vi "Calculate Intersection.vi"(0 "Coordinate Array":cluster{"X":dbl, "Y":dbl}[](array[cluster])=[{"X"=17.695146305622988, "Y"=13.693373640688556}, {"X"=17.43433821214924, "Y"=13.745589252995408}, {"X"=17.162615396419707, "Y"=13.800431502574536}, {"X"=16.880666961571364, "Y"=13.857854049761876}, {"X"=16.589182010741155, "Y"=13.917810554893407}, {"X"=16.288849647066037, "Y"=13.980254678305073}, {"X"=15.98035897368297, "Y"=14.045140080332846}, {"X"=15.664399093728898, "Y"=14.112420421312695}, {"X"=15.341659110340789, "Y"=14.182049361580557}, {"X"=15.012828126655597, "Y"=14.253980561472414}, {"X"=14.678595245810266, "Y"=14.328167681324217}, {"X"=14.339649570941765, "Y"=14.404564381471928}, {"X"=13.996680205187042, "Y"=14.483124322251506}, {"X"=13.650376251683053, "Y"=14.563801163998928}, {"X"=13.301426813566753, "Y"=14.646548567050132}, {"X"=12.950520993975104, "Y"=14.73132019174109}, {"X"=12.598347896045052, "Y"=14.818069698407761}, {"X"=12.245596622913556, "Y"=14.906750747386106}, {"X"=11.892956277717579, "Y"=14.997316999012082}, {"X"=11.541115963594061, "Y"=15.089722113621658}, {"X"=11.190764783679967, "Y"=15.183919751550793}, {"X"=10.842591841112258, "Y"=15.279863573135437}, {"X"=10.497286239027877, "Y"=15.377507238711566}, {"X"=10.155537080563787, "Y"=15.47680440861513}, {"X"=9.81803346885694, "Y"=15.577708743182097}, {"X"=9.485464507044295, "Y"=15.680173902748418}, {"X"=9.158519298262807, "Y"=15.78415354765006}, {"X"=8.837886945649426, "Y"=15.889601338222992}, {"X"=8.524256552341113, "Y"=15.99647093480316}, {"X"=8.21831722147482, "Y"=16.104715997726533}, {"X"=7.920758056187506, "Y"=16.21429018732907}, {"X"=7.6322681596161255, "Y"=16.325147163946735}, {"X"=7.3535366348976305, "Y"=16.437240587915483}, {"X"=7.0852525851689805, "Y"=16.55052411957128}, {"X"=6.82810511356713, "Y"=16.66495141925008}, {"X"=6.58278332322903, "Y"=16.78047614728785}, {"X"=6.3499763172916435, "Y"=16.89705196402055}, {"X"=6.13037319889192, "Y"=17.014632529784137}, {"X"=5.924663071166817, "Y"=17.13317150491458}, {"X"=5.733535037253291, "Y"=17.252622549747834}, {"X"=5.557678200288295, "Y"=17.372939324619853}, {"X"=5.397781663408787, "Y"=17.494075489866614}, {"X"=5.25453452975172, "Y"=17.61598470582406}, {"X"=5.128625902454051, "Y"=17.738620632828166}, {"X"=5.020744884652735, "Y"=17.861936931214885}], 1 "Enum":enum16{"Horizontal", "Vertical"}(ring), 3 "Vertical X":dbl=9.0, 4 "Horizontal Y":dbl=15.0) -> (5 "Intersection":bool=TRUE, 6 "Horizontal X":dbl=11.88266096329118, 7 "Vertical Y":dbl=15.83628649564717, 8 "XY Graph":cluster{dbl[], dbl[]}[](graph)=[{[5.020744884652735, 5.128625902454051, 5.25453452975172, 5.397781663408787, 5.557678200288295, 5.733535037253291, 5.924663071166817, 6.13037319889192, 6.3499763172916435, 6.58278332322903, 6.82810511356713, 7.0852525851689805, 7.3535366348976305, 7.6322681596161255, 7.920758056187506, 8.21831722147482, 8.524256552341113, 8.837886945649426, 9.158519298262807, 9.485464507044295, 9.81803346885694, 10.155537080563787, 10.497286239027877, 10.842591841112258, 11.190764783679967, 11.541115963594061, 11.892956277717579, 12.245596622913556, 12.598347896045052, 12.950520993975104, 13.301426813566753, 13.650376251683053, 13.996680205187042, 14.339649570941765, 14.678595245810266, 15.012828126655597, 15.341659110340789, 15.664399093728898, 15.98035897368297, 16.288849647066037, 16.589182010741155, 16.880666961571364, 17.162615396419707, 17.43433821214924, 17.695146305622988], [17.861936931214885, 17.738620632828166, 17.61598470582406, 17.494075489866614, 17.372939324619853, 17.252622549747834, 17.13317150491458, 17.014632529784137, 16.89705196402055, 16.78047614728785, 16.66495141925008, 16.55052411957128, 16.437240587915483, 16.325147163946735, 16.21429018732907, 16.104715997726533, 15.99647093480316, 15.889601338222992, 15.78415354765006, 15.680173902748418, 15.577708743182097, 15.47680440861513, 15.377507238711566, 15.279863573135437, 15.183919751550793, 15.089722113621658, 14.997316999012082, 14.906750747386106, 14.818069698407761, 14.73132019174109, 14.646548567050132, 14.563801163998928, 14.483124322251506, 14.404564381471928, 14.328167681324217, 14.253980561472414, 14.182049361580557, 14.112420421312695, 14.045140080332846, 13.980254678305073, 13.917810554893407, 13.857854049761876, 13.800431502574536, 13.745589252995408, 13.693373640688556]}, {[9.0, 9.0, 9.0, 9.0, 9.0, 9.0, 9.0, 9.0, 9.0, 9.0, 9.0, 9.0, 9.0, 9.0, 9.0, 9.0, 9.0, 9.0, 9.0, 9.0, 9.0, 9.0, 9.0, 9.0, 9.0, 9.0, 9.0, 9.0, 9.0, 9.0, 9.0, 9.0, 9.0, 9.0, 9.0, 9.0, 9.0, 9.0, 9.0, 9.0, 9.0, 9.0, 9.0, 9.0, 9.0], [17.861936931214885, 17.738620632828166, 17.61598470582406, 17.494075489866614, 17.372939324619853, 17.252622549747834, 17.13317150491458, 17.014632529784137, 16.89705196402055, 16.78047614728785, 16.66495141925008, 16.55052411957128, 16.437240587915483, 16.325147163946735, 16.21429018732907, 16.104715997726533, 15.99647093480316, 15.889601338222992, 15.78415354765006, 15.680173902748418, 15.577708743182097, 15.47680440861513, 15.377507238711566, 15.279863573135437, 15.183919751550793, 15.089722113621658, 14.997316999012082, 14.906750747386106, 14.818069698407761, 14.73132019174109, 14.646548567050132, 14.563801163998928, 14.483124322251506, 14.404564381471928, 14.328167681324217, 14.253980561472414, 14.182049361580557, 14.112420421312695, 14.045140080332846, 13.980254678305073, 13.917810554893407, 13.857854049761876, 13.800431502574536, 13.745589252995408, 13.693373640688556]}, {[9.0], [15.83628649564717]}])   [LabVIEW 2019]
doc: "This VI finds the interesection of a line with a set of coordinates."
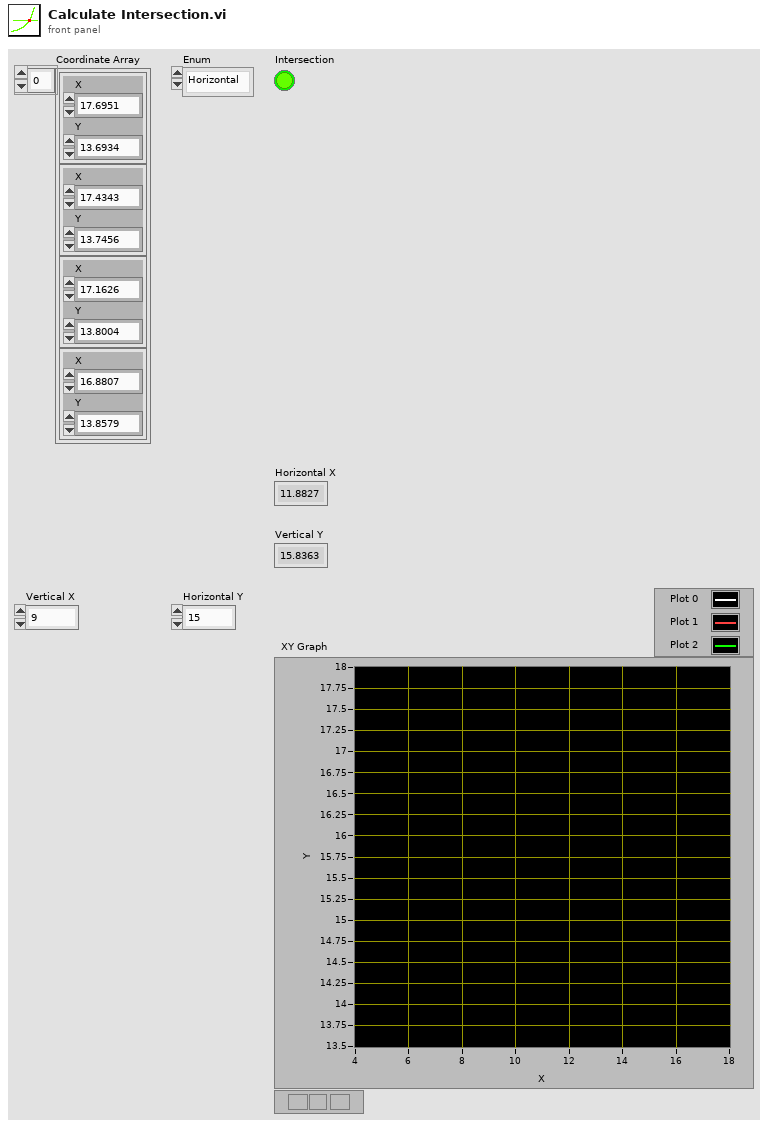
[diagram p1: front panel]
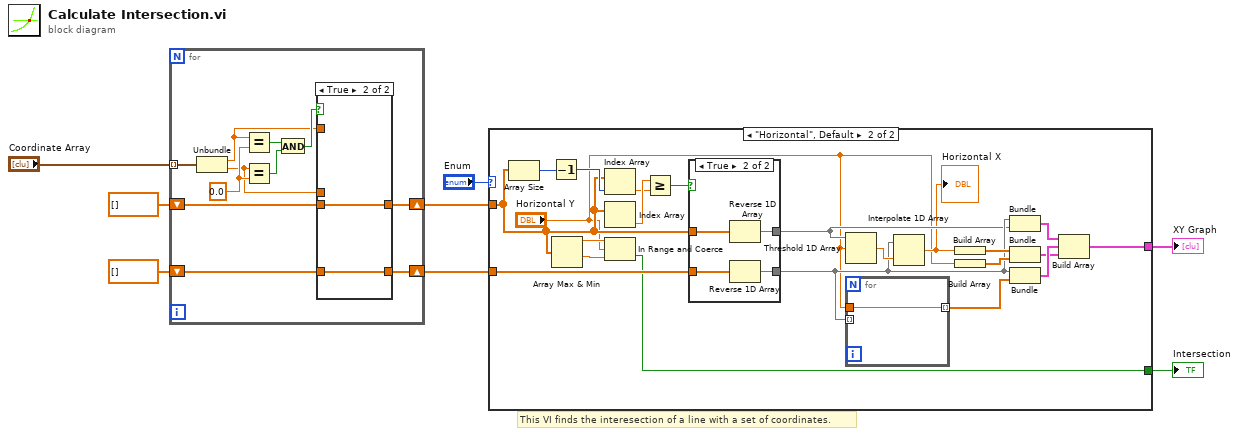
[diagram p0: block diagram]
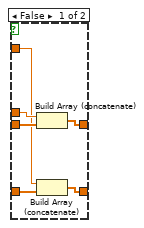
[diagram p2: hidden frame]
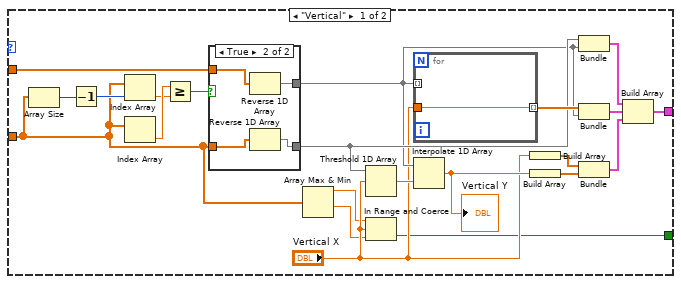
[diagram p3: hidden frame]
diagram:
  # "This VI finds the interesection of a line with a set of coordinates."
  n1 = for {
    tunnel: "Coordinate Array" -> [w19] mode=indexing
    shift-right: [w12] -> w2
    shift-left: dbl[] [] -> [w11]
    shift-right: [w10] -> w3
    shift-left: dbl[] [] -> [w9]
    w18 = 0.0 ("y")
    n2 = Unbundle(w19) -> ("X"=w14:dbl, "Y"=w13:dbl)
    n3 = Equal?(x=w14, y=w18) -> (x = y?=w17:bool)
    n4 = Equal?(x=w13, y=w18) -> (x = y?=w16:bool)
    n5 = And(x=w17, y=w16) -> (x .and. y?=w15:bool)
    n6 = case shown="True" w15 {
      tunnel: w14 -> [w22 _]
      tunnel: w13 -> [w25 _]
      tunnel: [w24 w27] -> w12
      tunnel: w11 -> [w23 w27]
      tunnel: [w21 w26] -> w10
      tunnel: w9 -> [w20 w26]
      frame False {
        n7 = Build Array (concatenate)(w25, w23) -> (w24:dbl[])
        n8 = Build Array (concatenate)(w22, w20) -> (w21:dbl[])
      }
      frame True {
      }
    }
  }
  n9 = case shown="\"Horizontal\", Default" "Enum" {
    tunnel: w2 -> [w36 w59]
    tunnel: w3 -> [w32 w65]
    tunnel: [w45 w72] -> w8
    tunnel: [w28 w57] -> w7
    frame "Vertical" {
      n10 = Array Size(array=w32) -> (size(s)=w41:i32)
      n11 = Decrement(x=w41) -> (x-1=w40:i32)
      n12 = Index Array(array=w32, index=w40) -> (element=w38:dbl)
      n13 = Index Array(array=w32) -> (element=w39:dbl)  [unwired: 1 in]
      n14 = Greater Or Equal?(x=w39, y=w38) -> (x >= y?=w37:bool)
      n15 = case shown="True" w37 {
        tunnel: w32 -> [w50 w55]
        tunnel: w36 -> [w51 w54]
        tunnel: [w50 w53] -> w35
        tunnel: [w51 w52] -> w34
        frame False {
        }
        frame True {
          n16 = Reverse 1D Array(array=w54) -> (reversed array=w52:dbl[])
          n17 = Reverse 1D Array(array=w55) -> (reversed array=w53:dbl[])
        }
      }
      n18 = Array Max & Min(array=w32) -> (max value=w30:dbl, min value=w29:dbl)  [unwired: 2 out]
      n19 = Threshold 1D Array(2:"Vertical X", 3:w35) -> (0:w49:dbl)  [unwired: 1 in]
      n20 = In Range and Coerce(upper limit=w30, x="Vertical X", lower limit=w29) -> (In Range?=w28:bool)  [unwired: 1 out]
      n21 = for {
        tunnel: w34 -> [_] mode=indexing
        tunnel: "Vertical X" -> [w56]
        tunnel: [w56] -> w42 mode=indexing
      }
      n22 = Interpolate 1D Array(1:w49, 2:w34) -> (0:w33:dbl)
      "Vertical Y" <- w33
      n23 = Build Array("Vertical X") -> (w44:dbl[])
      n24 = Build Array(w33) -> (w43:dbl[])
      n25 = Bundle(w35, w34) -> (w48:cluster{dbl[], dbl[]})  [unwired: 1 in]
      n26 = Bundle(w42, w34) -> (w47:cluster{dbl[], dbl[]})  [unwired: 1 in]
      n27 = Bundle(w44, w43) -> (w46:cluster{dbl[], dbl[]})  [unwired: 1 in]
      n28 = Build Array(w48, w47, w46) -> (w45:cluster{dbl[], dbl[]}[])
    }
    frame "Horizontal", Default {
      n29 = Array Size(array=w59) -> (size(s)=w70:i32)
      n30 = Decrement(x=w70) -> (x-1=w69:i32)
      n31 = Array Max & Min(array=w59) -> (max value=w61:dbl, min value=w60:dbl)  [unwired: 2 out]
      n32 = Index Array(array=w59, index=w69) -> (element=w67:dbl)
      n33 = Index Array(array=w59) -> (element=w68:dbl)  [unwired: 1 in]
      n34 = In Range and Coerce(upper limit=w61, x="Horizontal Y", lower limit=w60) -> (In Range?=w57:bool)  [unwired: 1 out]
      n35 = Greater Or Equal?(x=w68, y=w67) -> (x >= y?=w66:bool)
      n36 = case shown="True" w66 {
        tunnel: w65 -> [w79 w84]
        tunnel: w59 -> [w80 w83]
        tunnel: [w79 w82] -> w64
        tunnel: [w80 w81] -> w63
        frame False {
        }
        frame True {
          n37 = Reverse 1D Array(array=w83) -> (reversed array=w81:dbl[])
          n38 = Reverse 1D Array(array=w84) -> (reversed array=w82:dbl[])
        }
      }
      n39 = Threshold 1D Array(2:"Horizontal Y", 3:w63) -> (0:w78:dbl)  [unwired: 1 in]
      n40 = for {
        tunnel: w64 -> [_] mode=indexing
        tunnel: "Horizontal Y" -> [w85]
        tunnel: [w85] -> w77 mode=indexing
      }
      n41 = Interpolate 1D Array(1:w78, 2:w64) -> (0:w62:dbl)
      "Horizontal X" <- w62
      n42 = Build Array(w62) -> (w74:dbl[])
      n43 = Build Array("Horizontal Y") -> (w73:dbl[])
      n44 = Bundle(w64, w63) -> (w76:cluster{dbl[], dbl[]})  [unwired: 1 in]
      n45 = Bundle(w74, w73) -> (w71:cluster{dbl[], dbl[]})  [unwired: 1 in]
      n46 = Bundle(w64, w77) -> (w75:cluster{dbl[], dbl[]})  [unwired: 1 in]
      n47 = Build Array(w76, w75, w71) -> (w72:cluster{dbl[], dbl[]}[])
    }
  }
  "XY Graph" <- w8
  "Intersection" <- w7
